vi "Instrument Get Name.vi"(1 "Parameters":variant) -> (0 "Type":string)   [LabVIEW 2019]
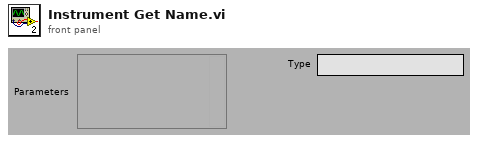
[diagram p1: front panel]
types:
  T1 = typedef "Private.ctl" = cluster{"Path":path, "VI Refnum":T2, "Name":string, "# of Values":i32, "Scale Factors":dbl[], "Display":T3[], "Offset":dbl[]}
  T2 = typedef "Instrument Ref.ctl" = refnum<vi>
  T3 = typedef "SystemCheckBox-resize.ctl" = bool
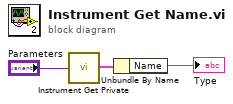
[diagram p0: block diagram]
diagram:
  n1 = call "Instrument Get Private.vi"("Variant"="Parameters") -> ("Private"=w3:T1)
  n2 = Unbundle By Name(w3) -> ("Name"=→"Type":string)
